vi "WAV_Convert.vi"(10 "data":waveform(dbl)[](array[waveform]), 11 "bit depth":u16=32) -> (0 "Data":waveform(sgl)[](graph), 2 "Data":sgl[][](array[numeric]), 3 "format":T1)   [LabVIEW 2022 SP3]
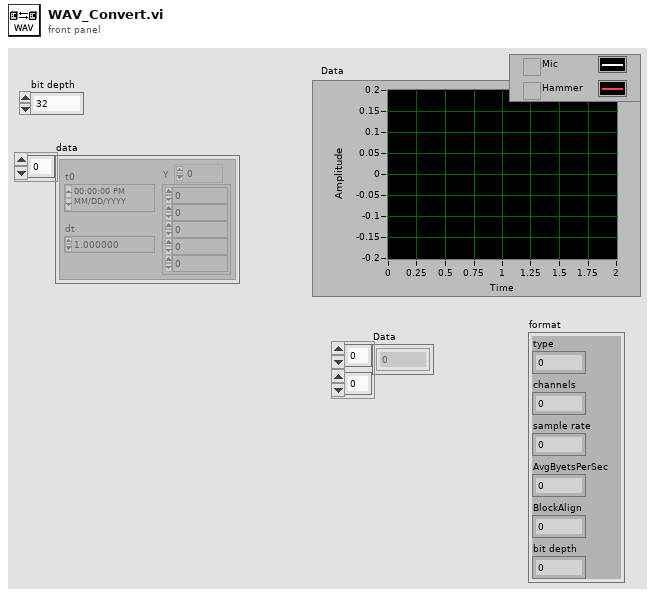
[diagram p1: front panel]
types:
  T1 = cluster{"type":u16, "channels":u16, "sample rate":u32, "AvgByetsPerSec":u32, "BlockAlign":u16, "bit depth":u16}
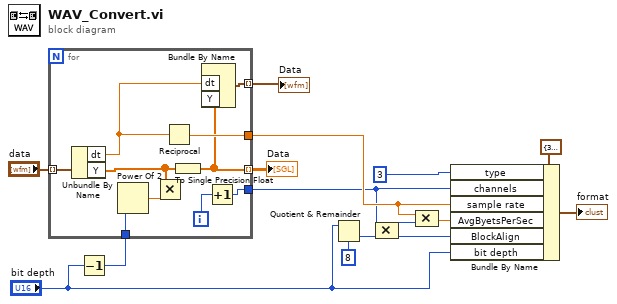
[diagram p0: block diagram]
diagram:
  n1 = Decrement(x="bit depth") -> (x-1=w13:u16)
  n2 = for {
    tunnel: "data" -> [w24] mode=indexing
    tunnel: [w16] -> w11 mode=indexing
    tunnel: [w22] -> w5
    tunnel: [w21] -> w14
    tunnel: w13 -> [w18]
    tunnel: [w15] -> w1 mode=indexing
    i -> [w23]
    n3 = Unbundle By Name(w24) -> ("dt"=w17:dbl, "Y"=w19:dbl[])
    n4 = Power Of 2(x=w18) -> (2^x=w20:dbl)
    n5 = Multiply(x=w19, y=w20) -> ()  [unwired: 1 out]
    n6 = Reciprocal(x=w17) -> (1/x=w21:dbl)
    n7 = To Single Precision Float(number=w19) -> (single precision float=w16:sgl[])
    n8 = Bundle By Name("dt"=w17, "Y"=w16) -> (w15:waveform(sgl))  [unwired: 1 in]
    n9 = Increment(x=w23) -> (x+1=w22:i32)
  }
  "Data" <- w1
  "Data" <- w11
  n10 = Quotient & Remainder(x="bit depth", y=u16 8 ("bit depth")) -> (floor(x/y)=w3:u16)  [unwired: 1 out]
  n11 = Compound Arithmetic op=MULTIPLY(w5, w3) -> (w6:i32)
  n12 = Compound Arithmetic op=MULTIPLY(w14, w6) -> (w7:dbl)
  n13 = Bundle By Name(cluster=T1 {"type"=3, "channels"=1, "sample rate"=44100, "AvgByetsPerSec"=176400, "BlockAlign"=4, "bit depth"=32} ("format"), "type"=u16 3, "channels"=w5, "sample rate"=w14, "AvgByetsPerSec"=w7, "BlockAlign"=w6, "bit depth"="bit depth") -> (→"format":T1)
